vi "WriteIO.a2dac.fpga.vi"(11 "Array":i16[](array[numeric])=[0, 0, 0, 0, 0, 0, 0, 0, 0, 0, 0, 0, 0, 0, 0, 0]) -> ()   [LabVIEW 2012]
uses:
  <vilib>/Platform/TimedLoop/XDataNode/timing_clust.ctl
  <vilib>/Platform/TimedLoop/XDataNode/nitl_modes.ctl
  <vilib>/Platform/TimedLoop/XDataNode/wakeup.ctl
  <vilib>/rvi/Emulation/niFpgaSctlEmulationRegisterWithScheduler.vi
  <vilib>/rvi/Emulation/niFpgaSctlEmulationScheduler.vi
  <vilib>/rvi/eio/common/nirviEmuTemplateMethod_errors.vi
  <vilib>/Platform/TimedLoop/XDataNode/XDataNode.xnode
  <vilib>/eio/EIONode/EIONode.xnode
  <vilib>/Platform/TimedLoop/XDataNode/XDNodeRunTimeDep.lvlib
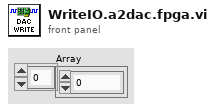
[diagram p1: front panel]
types:
  T1 = typedef "XDNodeRunTimeDep.lvlib/timing_clust.ctl" = cluster{"Expected End [f-1]":u64, "Actual End [f-1]":u64, "Finished Late? [f-1]":bool, "Expected End [i-1]":u64, "Actual End [i-1]":u64, "Finished Late? [i-1]":bool, "Expected Start [i]":u64, "Actual Start [i]":u64, "Expected Start [f]":u64, "Actual Start [f]":u64, "Source Name":string, "Structure Name":string, "Period":i64, "Deadline":i64, "Offset":i64, "Start":i64, "Priority":i32, "Timeout":i32, "Mode":T2, "Wakeup Reason":T3, "Error":errorcluster, "Source Type":string, "Secondary Source Type":string, "Global End Time":u64, "Global Start Time":u64, "Frame Duration":u64, "Iteration Duration":u64, "Assigned CPU":i32, "I/O Scan Engine Mode":u32}
  T2 = typedef "XDNodeRunTimeDep.lvlib/nitl_modes.ctl" = enum32{"No Change", "Process missed periods, maintain original phase", "Discard missed periods, maintain original phase", "Process missed periods, ignore original phase", "Discard missed periods, ignore original phase"}
  T3 = typedef "XDNodeRunTimeDep.lvlib/wakeup.ctl" = enum32{"Normal", "Aborted", "Asynchronous wakeup", "Timing source error", "Timed loop error", "Timeout"}
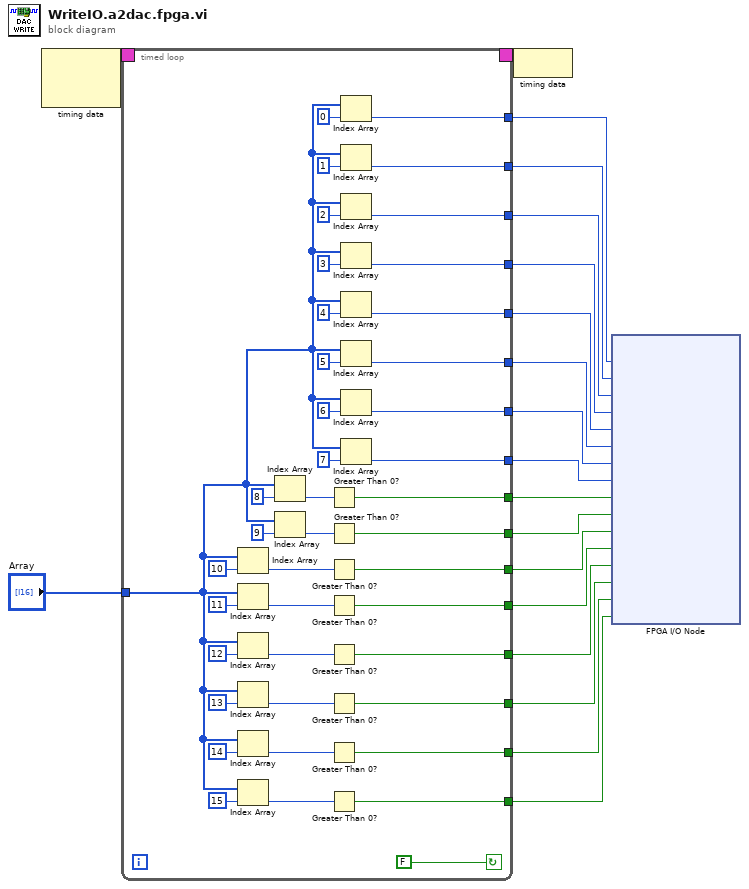
[diagram p0: block diagram]
diagram:
  n1 = node-c288() -> (w19:T1)  [unwired: 2 in]
  n2 = timed-loop {
    timing: w19 -> [_]
    timing-out: [_] -> w18
    tunnel: "Array" -> [w43]
    tunnel: [w61] -> w1
    tunnel: [w58] -> w2
    tunnel: [w42] -> w3
    tunnel: [w41] -> w4
    tunnel: [w40] -> w5
    tunnel: [w39] -> w6
    tunnel: [w38] -> w7
    tunnel: [w37] -> w8
    tunnel: [w36] -> w9
    tunnel: [w33] -> w10
    tunnel: [w31] -> w11
    tunnel: [w29] -> w12
    tunnel: [w27] -> w13
    tunnel: [w25] -> w14
    tunnel: [w23] -> w15
    tunnel: [w21] -> w16
    stop <- FALSE continue-if-true
    n3 = Index Array(array=w43, index=10) -> (element=w32:i16)
    n4 = Index Array(array=w43, index=11) -> (element=w30:i16)
    n5 = Index Array(array=w43, index=12) -> (element=w28:i16)
    n6 = Index Array(array=w43, index=13) -> (element=w26:i16)
    n7 = Index Array(array=w43, index=14) -> (element=w24:i16)
    n8 = Index Array(array=w43, index=15) -> (element=w22:i16)
    n9 = Index Array(array=w43, index=8) -> (element=w35:i16)
    n10 = Index Array(array=w43, index=9) -> (element=w34:i16)
    n11 = Greater Than 0?(x=w35) -> (x > 0?=w36:bool)
    n12 = Greater Than 0?(x=w34) -> (x > 0?=w33:bool)
    n13 = Greater Than 0?(x=w32) -> (x > 0?=w31:bool)
    n14 = Greater Than 0?(x=w30) -> (x > 0?=w29:bool)
    n15 = Greater Than 0?(x=w28) -> (x > 0?=w27:bool)
    n16 = Greater Than 0?(x=w26) -> (x > 0?=w25:bool)
    n17 = Greater Than 0?(x=w24) -> (x > 0?=w23:bool)
    n18 = Greater Than 0?(x=w22) -> (x > 0?=w21:bool)
    n19 = Index Array(array=w43, index=0) -> (element=w61:i16)
    n20 = Index Array(array=w43, index=1) -> (element=w58:i16)
    n21 = Index Array(array=w43, index=2) -> (element=w42:i16)
    n22 = Index Array(array=w43, index=3) -> (element=w41:i16)
    n23 = Index Array(array=w43, index=4) -> (element=w40:i16)
    n24 = Index Array(array=w43, index=5) -> (element=w39:i16)
    n25 = Index Array(array=w43, index=6) -> (element=w38:i16)
    n26 = Index Array(array=w43, index=7) -> (element=w37:i16)
  }
  n27 = node-c288(w18) -> ()
  n28 = xnode "FPGA I/O Node"("Connector0/AO0"=w1, "Connector0/AO1"=w2, "Connector0/AO2"=w3, "Connector0/AO3"=w4, "Connector0/AO4"=w5, "Connector0/AO5"=w6, "Connector0/AO6"=w7, "Connector0/AO7"=w8, "Connector0/DIO0"=w9, "Connector0/DIO1"=w10, "Connector0/DIO2"=w11, "Connector0/DIO3"=w12, "Connector0/DIO4"=w13, "Connector0/DIO5"=w14, "Connector0/DIO6"=w15, "Connector0/DIO7"=w16) -> ()  [unwired: 16 in, 16 out]
